vi "Output CRT Display.vi"(1 "Dark Pixel (.)":string=".", 3 "Register X":map{i32, i32}(c390), 4 "Lit Pixel (#)":string="#") -> (5 "CRT Display":string)   [LabVIEW 2020, in "AoC 2022.lvlib"]
uses:
  AoC 2022.lvlib
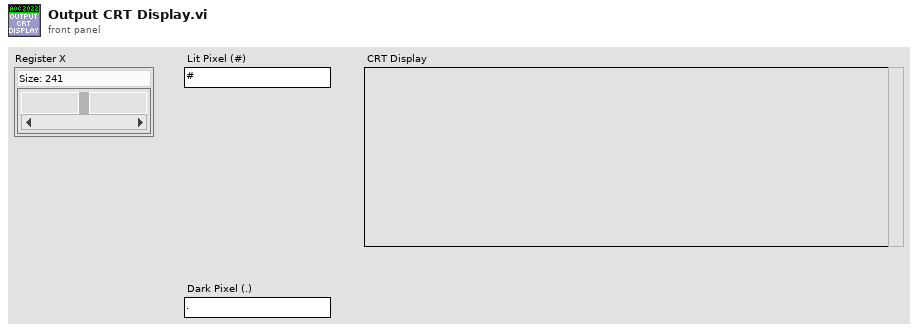
[diagram p1: front panel]
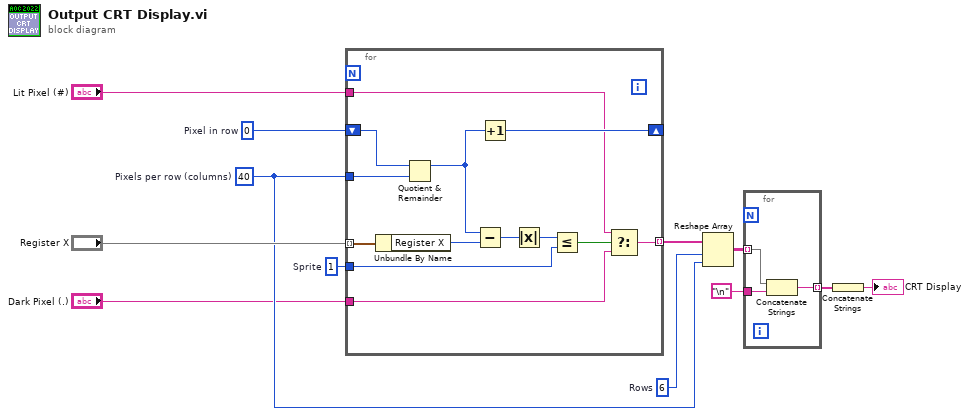
[diagram p0: block diagram]
diagram:
  w6 = 6  # Rows
  w12 = 1  # Sprite
  w3 = 0  # Pixel in row
  w5 = 40  # Pixels per row (columns)
  n1 = for {
    tunnel: "Register X" -> [w25] mode=indexing
    tunnel: w5 -> [w23]
    shift-right: [w22] -> _
    shift-left: w3 -> [w21]
    tunnel: w12 -> [w19]
    tunnel: [w17] -> w4 mode=indexing
    tunnel: "Lit Pixel (#)" -> [w14]
    tunnel: "Dark Pixel (.)" -> [w13]
    n2 = Unbundle By Name(w25) -> ("Register X"=w24:i32)
    n3 = Quotient & Remainder(x=w21, y=w23) -> (x-y*floor(x/y)=w15:i32)  [unwired: 1 out]
    n4 = Subtract(x=w15, y=w24) -> (x-y=w16:i32)
    n5 = Increment(x=w15) -> (x+1=w22:i32)
    n6 = Absolute Value(x=w16) -> (abs(x)=w20:i32)
    n7 = Less Or Equal?(x=w20, y=w19) -> (x <= y?=w18:bool)
    n8 = Select(t=w14, s=w18, f=w13) -> (s? t:f=w17:string)
  }
  n9 = Reshape Array(w4, w6, w5) -> (w8:string[][])
  n10 = for {
    tunnel: w8 -> [w28] mode=indexing
    tunnel: "\n" -> [w27]
    tunnel: [w26] -> w10 mode=indexing
    n11 = Concatenate Strings(w28, w27) -> (w26:string)
  }
  n12 = Concatenate Strings(w10) -> (→"CRT Display":string)
